vi "Exp_Test 1.vi"(0 "object in":refnum<class "SaveData.lvclass">, 1 "output cluster":T1, 4 "Oscilloscope Results":T2 {"Main Freq" format="%.2p"; "Main Volt" format="%.2p"}, 5 "error in (no error)":errorcluster) -> (14 "object out":refnum<class "SaveData.lvclass">, 19 "error out":errorcluster)   [LabVIEW 2023, in "SaveData.lvclass"]
uses:
  SaveData.lvclass
  <vilib>/express/express shared/transition.llb/Dynamic To Waveform Array.vi
  <vilib>/express/express signal manip/GetorSetDDTAttributes/Set DDT Attributes/SetT0.vi
  <vilib>/express/express shared/transition.llb/Waveform Array To Dynamic.vi
  <vilib>/express/express signal manip/GetorSetDDTAttributes/Set DDT Attributes/Set DDT Properties.xnode
  SaveData.lvclass/SaveData.ctl
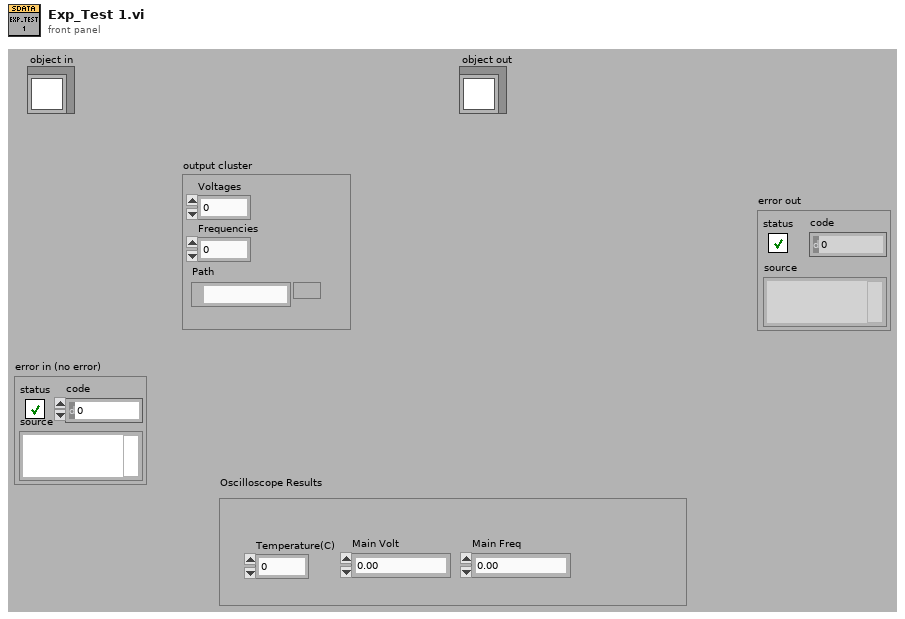
[diagram p1: front panel]
types:
  T1 = cluster{"Voltages":dbl, "Frequencies":dbl, "Path":path}
  T2 = cluster{"Main Volt":dbl, "Main Freq":dbl, "Temperature(C)":dbl}
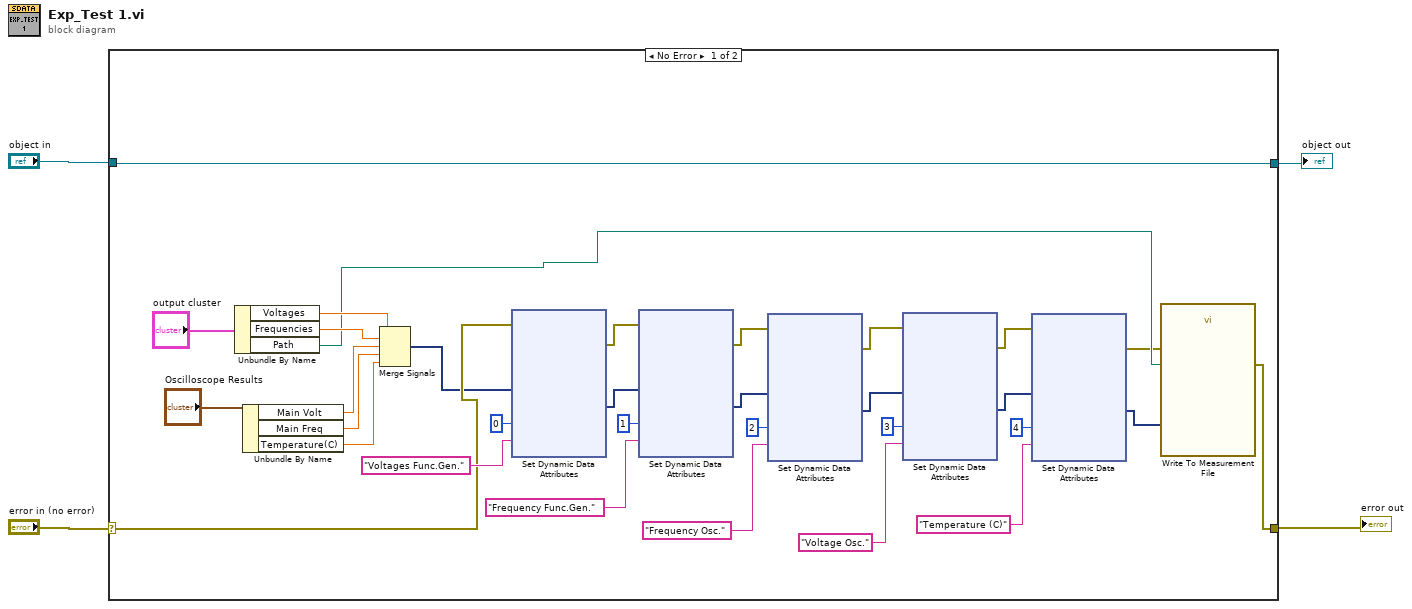
[diagram p0: block diagram]
diagram:
  n1 = case shown="No Error" "error in (no error)" {
    selector: "error in (no error)" -> [w30 w103]
    tunnel: [w29 w103] -> w3
    tunnel: [w28 w102] -> w1
    tunnel: "object in" -> [w28 w102]
    frame No Error {
      n2 = Unbundle By Name("output cluster") -> ("Voltages"=w17:dbl, "Frequencies"=w16:dbl, "Path"=w12:path)
      n3 = Unbundle By Name("Oscilloscope Results") -> ("Main Volt"=w15:dbl, "Main Freq"=w14:dbl, "Temperature(C)"=w11:dbl)
      n4 = Merge Signals(w17, w16, w15, w14, w11) -> (w13:dynamicdata)
      n5 = xnode "Set Dynamic Data Attributes"("Signals In"=w13, "Signal Index"=0, "Signal Name"="Voltages Func.Gen.", "error in"=w30) -> ("Signals Out"=w21:dynamicdata, "error out"=w33:errorcluster)
      n6 = xnode "Set Dynamic Data Attributes"("Signals In"=w21, "Signal Index"=1, "Signal Name"="Frequency Func.Gen.", "error in"=w33) -> ("Signals Out"=w20:dynamicdata, "error out"=w32:errorcluster)
      n7 = xnode "Set Dynamic Data Attributes"("Signals In"=w20, "Signal Index"=2, "Signal Name"="Frequency Osc.", "error in"=w32) -> ("Signals Out"=w19:dynamicdata, "error out"=w31:errorcluster)
      n8 = xnode "Set Dynamic Data Attributes"("Signals In"=w19, "Signal Index"=3, "Signal Name"="Voltage Osc.", "error in"=w31) -> ("Signals Out"=w9:dynamicdata, "error out"=w10:errorcluster)
      n9 = xnode "Set Dynamic Data Attributes"("Signals In"=w9, "Signal Index"=4, "Signal Name"="Temperature (C)", "error in"=w10) -> ("Signals Out"=w7:dynamicdata, "error out"=w6:errorcluster)
      n10 = call "Write To Measurement File"("Signals"=w7, "error in (no error)"=w6, "Filename"=w12) -> ("error out"=w29:errorcluster)  [unwired: 14 in, 2 out]
    }
    frame Error {
    }
  }
  "error out" <- w3
  "object out" <- w1
